vi "Contour plot test.vi"() -> ()   [LabVIEW 2018]
uses:
  <vilib>/Native 3D Graph/xcontrol/3DPC_SurfacePlot.xctl
  <vilib>/Math Plots/3D Math Plots/3D Surface/3D Surface XCtrl/3D Surface.xctl
  <vilib>/Math Plots/3D Math Plots/3D Contour/3D Contour XCtrl/3D Contour.xctl
  <vilib>/Heliosphere Research LLC/Advanced Plotting Toolkit/api_core/NewPlotProperties.ctl
  <vilib>/Heliosphere Research LLC/Advanced Plotting Toolkit/typedefs/PlotColor.ctl
  <vilib>/Heliosphere Research LLC/Advanced Plotting Toolkit/api_plotting/ContourProperties.ctl
  <vilib>/Heliosphere Research LLC/Advanced Plotting Toolkit/properties/Line.ctl
  <vilib>/Heliosphere Research LLC/Advanced Plotting Toolkit/properties/Line_Style.ctl
  <vilib>/Heliosphere Research LLC/Advanced Plotting Toolkit/properties/Display.ctl
  <vilib>/Heliosphere Research LLC/Advanced Plotting Toolkit/api_plotting/ArrayViewBoundaries.ctl
  <vilib>/Heliosphere Research LLC/Advanced Plotting Toolkit/api_plotting/ArrayViewProperties.ctl
  <vilib>/Heliosphere Research LLC/Advanced Plotting Toolkit/properties/Colormap.ctl
  <vilib>/Heliosphere Research LLC/Advanced Plotting Toolkit/properties/Colormap_Map.ctl
  <vilib>/Heliosphere Research LLC/Advanced Plotting Toolkit/properties/Colormap_Scaling.ctl
  <vilib>/Heliosphere Research LLC/Advanced Plotting Toolkit/api_core/NewPlotType.ctl
  <vilib>/Heliosphere Research LLC/Advanced Plotting Toolkit/api_core/NewPlotScales.ctl
  <vilib>/Heliosphere Research LLC/Advanced Plotting Toolkit/api_plotting/Contour_Automatic.vi
  <vilib>/express/express arith-compare/Formula/XNode/ExpressFormulaBlockNode.xnode
  <vilib>/Heliosphere Research LLC/Advanced Plotting Toolkit/Advanced Plotting Toolkit.lvlib
  <vilib>/Heliosphere Research LLC/Advanced Plotting Toolkit/api_plotting/ContourFilled_Automatic.vi
  <vilib>/Analysis/NI_AAL_Geometry.lvlib
  <vilib>/Analysis/geometry.llb/Contour Line (Number of Heights).vi
  <vilib>/Math Plots/3D Math Plots/3D Surface/3D Surface Datatype/3D Surface Datatype.lvclass
  <vilib>/Math Plots/3D Math Plots/3D Surface/3D Surface Datatype/Public/Plot Helper (Vector).vi
  <vilib>/Math Plots/3D Math Plots/3D Contour/3D Contour Datatype/3D Contour Datatype.lvclass
  <vilib>/Math Plots/3D Math Plots/3D Contour/3D Contour Datatype/Public/Plot Helper (Vector).vi
panel:
  in  "View Array properties":T1={"Colormap"={"Map"=enum."Automatic", "Value Min"=nan, "Value Max"=nan, "Scaling"=enum."Default", "Reverse"=FALSE}, "Display"={"Alpha"=nan, "Z Order"=nan}}
  in  "View Array Boundaries":T6={"X Min"=-2.0, "X Max"=2.0, "Y Min"=-2.0, "Y Max"=2.0}
  in  "Countors Properties":T7={"Label Contours"=TRUE, "Line"={"Style"=enum."Automatic", "Color"=2147483647, "Width"=nan}, "Display"={"Alpha"=nan, "Z Order"=nan}} {"Line"."Color" items=["Automatic"=2147483647, "Black"=0, "White"=16777215, "Red"=16711680, "Green"=2263842, "Blue"=255, "Cyan"=65535, "Magenta"=16711935, "Yellow"=16776960]}
  in  "Plot Properties":T11={"Background Color"=2147483647, "Axis Background"=2147483647, "Left Margin"=nan, "Right Margin"=nan, "Bottom Margin"=nan, "Top Margin"=nan, "Aspect Ratio"=nan} {"Axis Background" items=["Automatic"=2147483647, "Black"=0, "White"=16777215, "Red"=16711680, "Green"=2263842, "Blue"=255, "Cyan"=65535, "Magenta"=16711935, "Yellow"=16776960]; "Background Color" items=["Automatic"=2147483647, "Black"=0, "White"=16777215, "Red"=16711680, "Green"=2263842, "Blue"=255, "Cyan"=65535, "Magenta"=16711935, "Yellow"=16776960]}
  out "error out":errorcluster
  out "Picture":picture
  out "3D Contour":refnum<class "3D Plot Datatype.lvclass">[](xcontrol)
  out "3D Surface":refnum<class "3D Plot Datatype.lvclass">[](xcontrol)
  out "3D Graph":refnum<class "Base Datatype.lvclass">[](xcontrol)
  out "XY Graph":cluster{dbl[], dbl[]}[](graph)
  out "Array 3":dbl[](array[numeric])
  out "Array 2":dbl[](array[numeric])
  out "Array":dbl[](array[numeric])
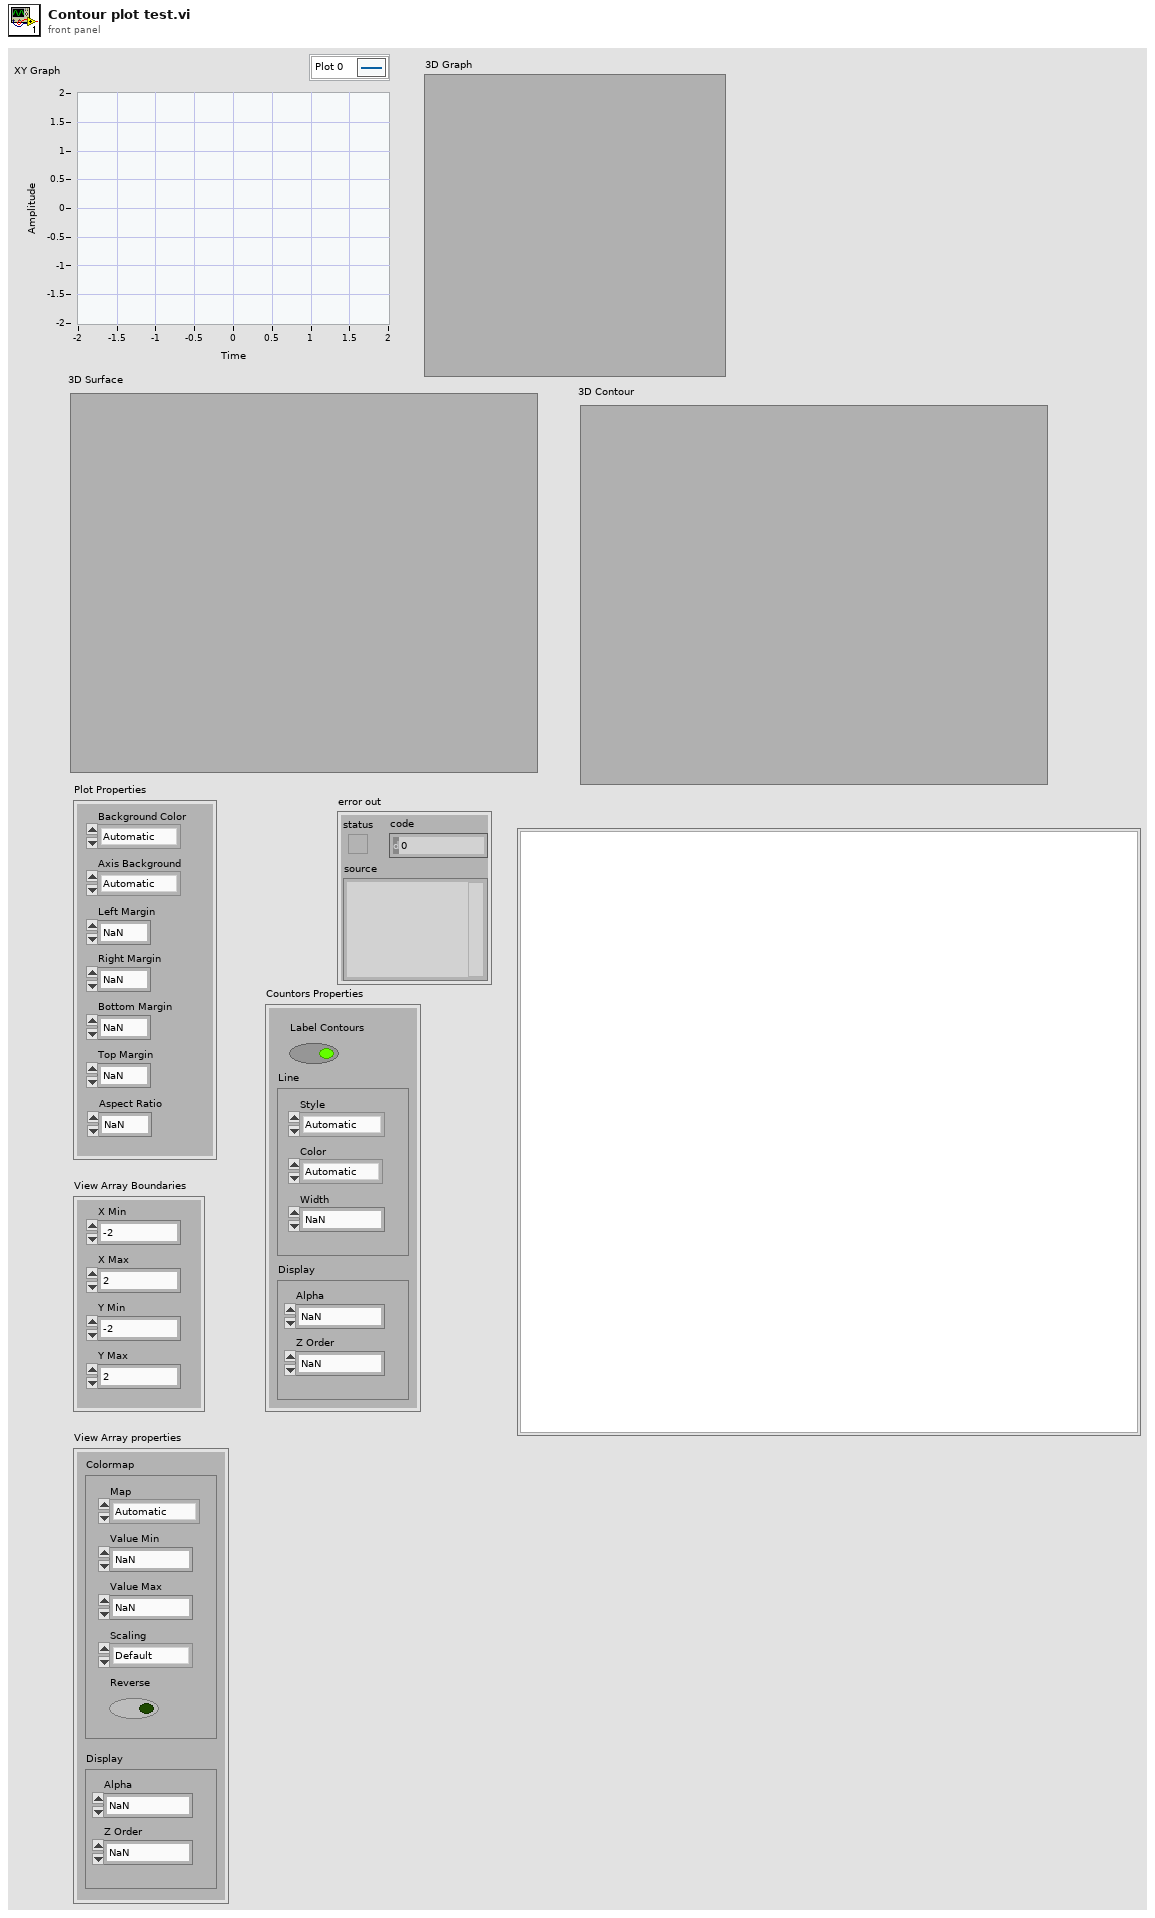
[diagram p1: front panel]
types:
  T1 = typedef "Advanced Plotting Toolkit.lvlib/ArrayViewProperties.ctl" = cluster{"Colormap":T2, "Display":T5}
  T2 = typedef "Advanced Plotting Toolkit.lvlib/Colormap.ctl" = cluster{"Map":T3, "Value Min":dbl, "Value Max":dbl, "Scaling":T4, "Reverse":bool}
  T3 = typedef "Advanced Plotting Toolkit.lvlib/Colormap_Map.ctl" = enum16{"Automatic", "Rainbow", "Hot and Cold", "White-Black", "White-Blue", "White-Green", "White-Red", "Fire", "Water", "Earth", "Air", "Pastel", "Banded", "Stepped"}
  T4 = typedef "Advanced Plotting Toolkit.lvlib/Colormap_Scaling.ctl" = enum16{"Default"}
  T5 = typedef "Advanced Plotting Toolkit.lvlib/Display.ctl" = cluster{"Alpha":dbl, "Z Order":dbl}
  T6 = typedef "Advanced Plotting Toolkit.lvlib/ArrayViewBoundaries.ctl" = cluster{"X Min":dbl, "X Max":dbl, "Y Min":dbl, "Y Max":dbl}
  T7 = typedef "Advanced Plotting Toolkit.lvlib/ContourProperties.ctl" = cluster{"Label Contours":bool, "Line":T8, "Display":T5}
  T8 = typedef "Advanced Plotting Toolkit.lvlib/Line.ctl" = cluster{"Style":T9, "Color":T10, "Width":sgl}
  T9 = typedef "Advanced Plotting Toolkit.lvlib/Line_Style.ctl" = enum16{"Automatic", "Solid", "Dashed", "Dotted", "Dash-dot", "Invisible"}
  T10 = typedef "Advanced Plotting Toolkit.lvlib/PlotColor.ctl" = u32
  T11 = typedef "Advanced Plotting Toolkit.lvlib/NewPlotProperties.ctl" = cluster{"Background Color":T10, "Axis Background":T10, "Left Margin":dbl, "Right Margin":dbl, "Bottom Margin":dbl, "Top Margin":dbl, "Aspect Ratio":dbl}
  T12 = typedef "Advanced Plotting Toolkit.lvlib/NewPlotScales.ctl" = enum16{"Default", "Linear", "Log", "Symlog"}
  T13 = typedef "Advanced Plotting Toolkit.lvlib/NewPlotType.ctl" = enum16{"Rectangular Axes", "Polar Axes"}
  T14 = typedef "Advanced Plotting Toolkit.lvlib/PlotID.ctl" = i32
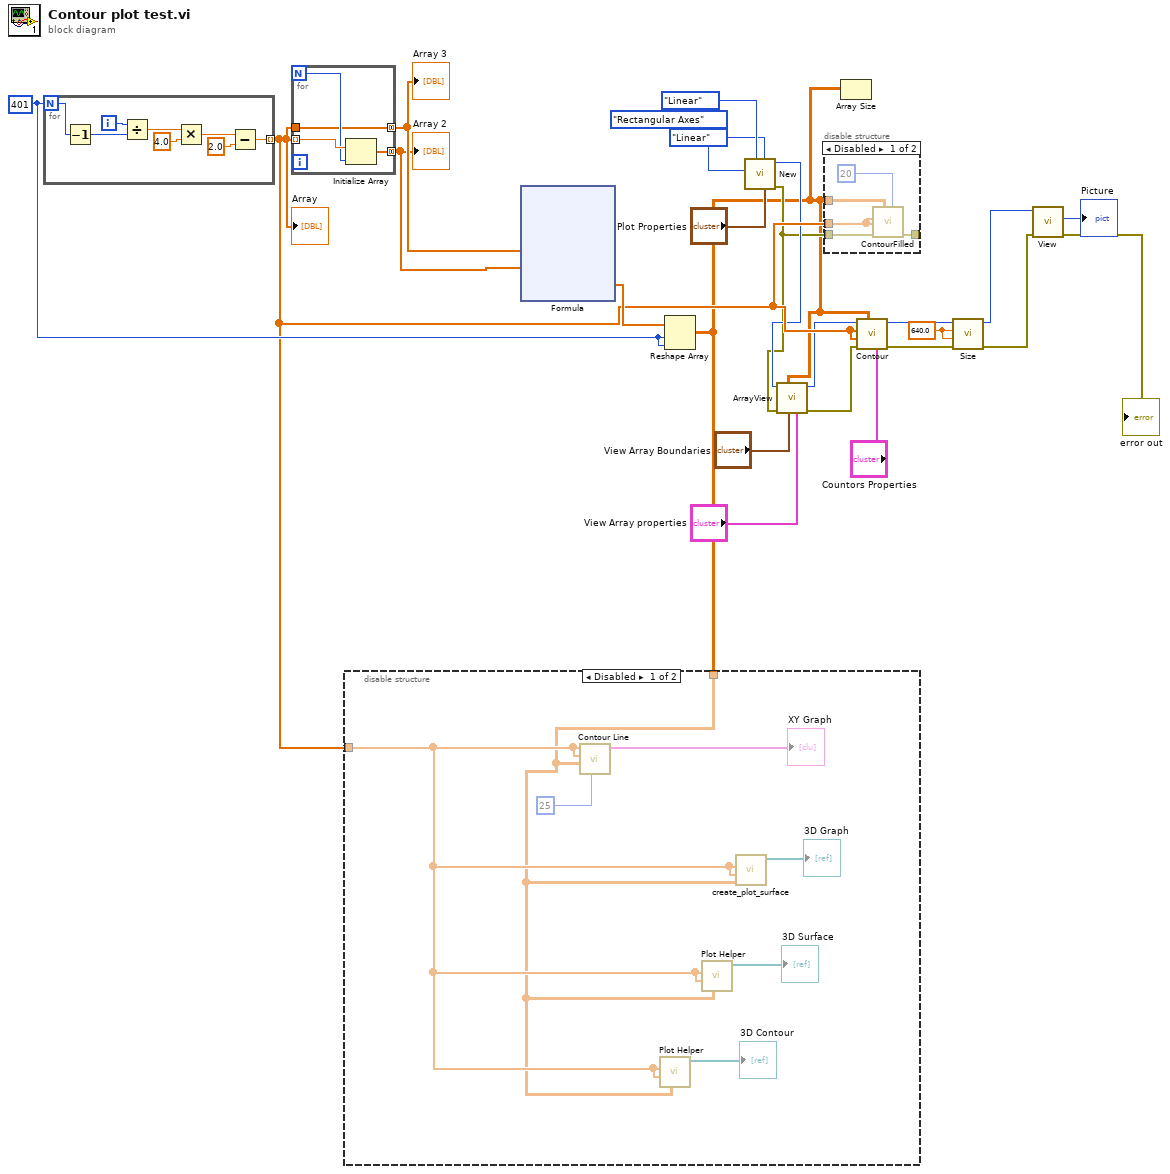
[diagram p0: block diagram]
diagram:
  w1 = 640.0 ("Width (pixels)")
  w24 = 401
  n1 = for {
    N: w24 -> [w32]
    tunnel: [w25] -> w14 mode=indexing
    i -> [w27]
    n2 = Decrement(x=w32) -> (x-1=w26:i32)
    n3 = Divide(x=w27, y=w26) -> (x/y=w28:dbl)
    n4 = Multiply(x=w28, y=4.0) -> (x*y=w30:dbl)
    n5 = Subtract(x=w30, y=2.0) -> (x-y=w25:dbl)
  }
  "Array" <- w14
  n6 = for {
    N -> [w35]
    tunnel: w14 -> [w36] mode=indexing
    tunnel: [w34] -> w21 mode=concatenating
    tunnel: w14 -> [w33]
    tunnel: [w33] -> w22 mode=concatenating
    n7 = Initialize Array(w36, w35) -> (w34:dbl[])
  }
  "Array 2" <- w21
  "Array 3" <- w22
  n8 = xnode "Formula"("X"=w22, "Y"=w21) -> ("Result"=w19:dbl[])  [unwired: 1 in, 1 out]
  n9 = Reshape Array(w19, w24, w24) -> (w6:dbl[][])
  n10 = disable-structure shown="Disabled" {
    disable-tunnel: w14 -> [w43 _]
    disable-tunnel: w6 -> [w42 _]
    frame Disabled {
      n11 = call-poly <vilib>:"Contour Line.vi"("number of heights"=25, "Z"=w42, "Y"=w43, "X"=w43) -> ("Contour Graph"=→"XY Graph":cluster{dbl[], dbl[]}[])  [unwired: 5 in, 2 out]
      n12 = call-poly <vilib>:"Plot Helper.vi"("z matrix"=w42, "y vector"=w43, "x vector"=w43) -> ("3D Plot lvclass Array out"=→"3D Contour":refnum<class "3D Plot Datatype.lvclass">[])  [unwired: 3 in, 5 out]
      n13 = call-poly <vilib>:"Plot Helper.vi"("z matrix"=w42, "y vector"=w43, "x vector"=w43) -> ("3D Plot lvclass Array out"=→"3D Surface":refnum<class "3D Plot Datatype.lvclass">[])  [unwired: 3 in, 5 out]
      n14 = call <vilib>:"create_plot_surface.vi"("z matrix"=w42, "y vector"=w43, "x vector"=w43) -> ("plots out"=→"3D Graph":refnum<class "Base Datatype.lvclass">[])  [unwired: 2 in, 6 out]
    }
    frame Enabled {
    }
  }
  n15 = call <vilib>:"New.vi"("Properties"="Plot Properties", "Y Axis Scale"=NewPlotScales."Linear", "X Axis Scale"=NewPlotScales."Linear", "Plot Type"=NewPlotType."Rectangular Axes") -> ("error out"=w10:errorcluster, "Plot ID"=w12:T14)  [unwired: 6 in]
  n16 = call <vilib>:"ArrayView.vi"("Properties"="View Array properties", "Boundaries"="View Array Boundaries", "Data"=w6, "error in (no error)"=w10, "Plot ID"=w12) -> ("error out"=w9:errorcluster, "Plot ID Out"=w11:T14)  [unwired: 5 in]
  n17 = disable-structure shown="Disabled" {
    disable-tunnel: w6 -> [w48 _]
    disable-tunnel: w14 -> [w47 _]
    disable-tunnel: [w46 _] -> _
    disable-tunnel: w10 -> [w44 _]
    frame Disabled {
      n18 = call-poly <vilib>:"ContourFilled.vi"("Levels"=20, "Z Data"=w48, "error in (no error)"=w44, "Y Coordinates"=w47, "X Coordinates"=w47) -> ("error out"=w46:errorcluster)  [unwired: 5 in, 1 out]
    }
    frame Enabled {
    }
  }
  n19 = Array Size(array=w6) -> ()  [unwired: 1 out]
  n20 = call-poly <vilib>:"Contour.vi"("Properties"="Countors Properties", "Z Data"=w6, "error in (no error)"=w9, "Y Coordinates"=w14, "X Coordinates"=w14, "Plot ID"=w11) -> ("error out"=w5:errorcluster, "Plot ID Out"=w4:T14)  [unwired: 4 in]
  n21 = call <vilib>:"Size.vi"("error in (no error)"=w5, "Height (pixels)"=w1, "Width (pixels)"=w1, "Plot ID"=w4) -> ("error out"=w2:errorcluster, "Plot ID Out"=w3:T14)  [unwired: 6 in]
  n22 = call <vilib>:"View.vi"("error in (no error)"=w2, "Plot ID"=w3) -> ("error out"=→"error out":errorcluster, "Picture"=→"Picture":picture)  [unwired: 7 in, 1 out]
